vi "Methods_Insert Dividers.vi"(11 "Methods[] In":T1(array[cluster])) -> (3 "Methods[] Out":T1(array[cluster]))   [LabVIEW 2023] (continued)
name (localized)"="Convert To FlatSeq", "Long name (localized)"="Convert To Flat Sequence"}, "Method Flags"={"IsDeprecated"=FALSE, "IsPrivate"=FALSE, "IsScripting"=TRUE, "IsNotInRun-Time"=FALSE}, "Divider"=FALSE}, {"Class Info"={"Unique ID string"="16408", "Parent ID string"="16406", "Class Name (unlocalized)"="CaseStructure", "Class Name (localized)"="CaseStructure"}, "Method Info"={"Unique ID string"="6364c00", "Data name"="Remove Empty Cases", "Short name (localized)"="Remove Empty Cases", "Long name (localized)"="Remove Empty Cases"}, "Method Flags"={"IsDeprecated"=FALSE, "IsPrivate"=FALSE, "IsScripting"=TRUE, "IsNotInRun-Time"=TRUE}, "Divider"=FALSE}, {"Class Info"={"Unique ID string"="16408", "Parent ID string"="16406", "Class Name (unlocalized)"="CaseStructure", "Class Name (localized)"="CaseStructure"}, "Method Info"={"Unique ID string"="6364c02", "Data name"="SetDefaultCase", "Short name (localized)"="SetDefaultCase", "Long name (localized)"="Set Default Case"}, "Method Flags"={"IsDeprecated"=FALSE, "IsPrivate"=FALSE, "IsScripting"=TRUE, "IsNotInRun-Time"=TRUE}, "Divider"=FALSE}, {"Class Info"={"Unique ID string"="16408", "Parent ID string"="16406", "Class Name (unlocalized)"="CaseStructure", "Class Name (localized)"="CaseStructure"}, "Method Info"={"Unique ID string"="6364c03", "Data name"="RemoveDefault", "Short name (localized)"="RemoveDefault", "Long name (localized)"="Remove Default"}, "Method Flags"={"IsDeprecated"=FALSE, "IsPrivate"=FALSE, "IsScripting"=TRUE, "IsNotInRun-Time"=TRUE}, "Divider"=FALSE}, {"Class Info"={"Unique ID string"="16408", "Parent ID string"="16406", "Class Name (unlocalized)"="CaseStructure", "Class Name (localized)"="CaseStructure"}, "Method Info"={"Unique ID string"="6364c04", "Data name"="GetFrameIndex", "Short name (localized)"="GetFrameIndex", "Long name (localized)"="Get Frame Index"}, "Method Flags"={"IsDeprecated"=FALSE, "IsPrivate"=FALSE, "IsScripting"=TRUE, "IsNotInRun-Time"=FALSE}, "Divider"=FALSE}, {"Class Info"={"Unique ID string"="16409", "Parent ID string"="16421", "Class Name (unlocalized)"="Formula", "Class Name (localized)"="Formula"}, "Method Info"={"Unique ID string"="6365800", "Data name"="Add Input", "Short name (localized)"="Add Input", "Long name (localized)"="Add Input"}, "Method Flags"={"IsDeprecated"=FALSE, "IsPrivate"=FALSE, "IsScripting"=TRUE, "IsNotInRun-Time"=TRUE}, "Divider"=FALSE}, {"Class Info"={"Unique ID string"="16409", "Parent ID string"="16421", "Class Name (unlocalized)"="Formula", "Class Name (localized)"="Formula"}, "Method Info"={"Unique ID string"="6365801", "Data name"="Add Output", "Short name (localized)"="Add Output", "Long name (localized)"="Add Output"}, "Method Flags"={"IsDeprecated"=FALSE, "IsPrivate"=FALSE, "IsScripting"=TRUE, "IsNotInRun-Time"=TRUE}, "Divider"=FALSE}, {"Class Info"={"Unique ID string"="16410", "Parent ID string"="16421", "Class Name (unlocalized)"="GrowableFunction", "Class Name (localized)"="GrowableFunction"}, "Method Info"={"Unique ID string"="6367c01", "Data name"="Resize.AddChunk", "Short name (localized)"="Resize.AddChunk", "Long name (localized)"="Resize:Add Chunk"}, "Method Flags"={"IsDeprecated"=FALSE, "IsPrivate"=FALSE, "IsScripting"=TRUE, "IsNotInRun-Time"=TRUE}, "Divider"=FALSE}, {"Class Info"={"Unique ID string"="16410", "Parent ID string"="16421", "Class Name (unlocalized)"="GrowableFunction", "Class Name (localized)"="GrowableFunction"}, "Method Info"={"Unique ID string"="6367c02", "Data name"="Resize.RemoveChunk", "Short name (localized)"="Resize.RemoveChunk", "Long name (localized)"="Resize:Remove Chunk"}, "Method Flags"={"IsDeprecated"=FALSE, "IsPrivate"=FALSE, "IsScripting"=TRUE, "IsNotInRun-Time"=TRUE}, "Divider"=FALSE}, {"Class Info"={"Unique ID string"="16416", "Parent ID string"="16410", "Class Name (unlocalized)"="CIN", "Class Name (localized)"="CIN"}, "Method Info"={"Unique ID string"="636c400", "Data name"="Load Code Resource", "Short name (localized)"="Load Code Resource", "Long name (localized)"="Load Code Resource"}, "Method Flags"={"IsDeprecated"=FALSE, "IsPrivate"=FALSE, "IsScripting"=TRUE, "IsNotInRun-Time"=TRUE}, "Divider"=FALSE}, {"Class Info"={"Unique ID string"="16416", "Parent ID string"="16410", "Class Name (unlocalized)"="CIN", "Class Name (localized)"="CIN"}, "Method Info"={"Unique ID string"="636c401", "Data name"="Create C File", "Short name (localized)"="Create C File", "Long name (localized)"="Create C File"}, "Method Flags"={"IsDeprecated"=FALSE, "IsPrivate"=FALSE, "IsScripting"=TRUE, "IsNotInRun-Time"=TRUE}, "Divider"=FALSE}, {"Class Info"={"Unique ID string"="16416", "Parent ID string"="16410", "Class Name (unlocalized)"="CIN", "Class Name (localized)"="CIN"}, "Method Info"={"Unique ID string"="636c402", "Data name"="AddParameterAfter", "Short name (localized)"="AddParameterAfter", "Long name (localized)"="Add Parameter After"}, "Method Flags"={"IsDeprecated"=FALSE, "IsPrivate"=FALSE, "IsScripting"=TRUE, "IsNotInRun-Time"=FALSE}, "Divider"=FALSE}, {"Class Info"={"Unique ID string"="16416", "Parent ID string"="16410", "Class Name (unlocalized)"="CIN", "Class Name (localized)"="CIN"}, "Method Info"={"Unique ID string"="636c403", "Data name"="RemoveParameter", "Short name (localized)"="RemoveParameter", "Long name (localized)"="Remove Parameter"}, "Method Flags"={"IsDeprecated"=FALSE, "IsPrivate"=FALSE, "IsScripting"=TRUE, "IsNotInRun-Time"=FALSE}, "Divider"=FALSE}, {"Class Info"={"Unique ID string"="16416", "Parent ID string"="16410", "Class Name (unlocalized)"="CIN", "Class Name (localized)"="CIN"}, "Method Info"={"Unique ID string"="636c404", "Data name"="PurgeCodeResource", "Short name (localized)"="PurgeCodeResource", "Long name (localized)"="Purge Code Resource"}, "Method Flags"={"IsDeprecated"=FALSE, "IsPrivate"=FALSE, "IsScripting"=TRUE, "IsNotInRun-Time"=FALSE}, "Divider"=FALSE}, {"Class Info"={"Unique ID string"="16417", "Parent ID string"="16410", "Class Name (unlocalized)"="CallLibrary", "Class Name (localized)"="CallLibrary"}, "Method Info"={"Unique ID string"="636d000", "Data name"="Prototype", "Short name (localized)"="Prototype", "Long name (localized)"="Prototype"}, "Method Flags"={"IsDeprecated"=FALSE, "IsPrivate"=FALSE, "IsScripting"=TRUE, "IsNotInRun-Time"=TRUE}, "Divider"=FALSE}, {"Class Info"={"Unique ID string"="16417", "Parent ID string"="16410", "Class Name (unlocalized)"="CallLibrary", "Class Name (localized)"="CallLibrary"}, "Method Info"={"Unique ID string"="636d001", "Data name"="CreateCFile", "Short name (localized)"="CreateCFile", "Long name (localized)"="Create C File"}, "Method Flags"={"IsDeprecated"=FALSE, "IsPrivate"=FALSE, "IsScripting"=TRUE, "IsNotInRun-Time"=FALSE}, "Divider"=FALSE}, {"Class Info"={"Unique ID string"="16417", "Parent ID string"="16410", "Class Name (unlocalized)"="CallLibrary", "Class Name (localized)"="CallLibrary"}, "Method Info"={"Unique ID string"="636d002", "Data name"="TypeOnlyParam", "Short name (localized)"="TypeOnlyParam", "Long name (localized)"="Type Only Param"}, "Method Flags"={"IsDeprecated"=FALSE, "IsPrivate"=TRUE, "IsScripting"=TRUE, "IsNotInRun-Time"=FALSE}, "Divider"=FALSE}, {"Class Info"={"Unique ID string"="16419", "Parent ID string"="16418", "Class Name (unlocalized)"="Property", "Class Name (localized)"="Property"}, "Method Info"={"Unique ID string"="636f400", "Data name"="Get Prop Item", "Short name (localized)"="Get Prop Item", "Long name (localized)"="Get Property Item"}, "Method Flags"={"IsDeprecated"=FALSE, "IsPrivate"=FALSE, "IsScripting"=TRUE, "IsNotInRun-Time"=TRUE}, "Divider"=FALSE}, {"Class Info"={"Unique ID string"="16419", "Parent ID string"="16418", "Class Name (unlocalized)"="Property", "Class Name (localized)"="Property"}, "Method Info"={"Unique ID string"="636f401", "Data name"="AddPropertyItemAfter", "Short name (localized)"="AddPropertyItemAfter", "Long name (localized)"="Add Property Item After"}, "Method Flags"={"IsDeprecated"=FALSE, "IsPrivate"=FALSE, "IsScripting"=TRUE, "IsNotInRun-Time"=FALSE}, "Divider"=FALSE}, {"Class Info"={"Unique ID string"="16419", "Parent ID string"="16418", "Class Name (unlocalized)"="Property", "Class Name (localized)"="Property"}, "Method Info"={"Unique ID string"="636f402", "Data name"="RemovePropertyItem", "Short name (localized)"="RemovePropertyItem", "Long name (localized)"="Remove Property Item"}, "Method Flags"={"IsDeprecated"=FALSE, "IsPrivate"=FALSE, "IsScripting"=TRUE, "IsNotInRun-Time"=FALSE}, "Divider"=FALSE}, {"Class Info"={"Unique ID string"="16419", "Parent ID string"="16418", "Class Name (unlocalized)"="Property", "Class Name (localized)"="Property"}, "Method Info"={"Unique ID string"="636f403", "Data name"="LinkToControl", "Short name (localized)"="LinkToControl", "Long name (localized)"="Link To Control"}, "Method Flags"={"IsDeprecated"=FALSE, "IsPrivate"=FALSE, "IsScripting"=TRUE, "IsNotInRun-Time"=FALSE}, "Divider"=FALSE}, {"Class Info"={"Unique ID string"="16419", "Parent ID string"="16418", "Class Name (unlocalized)"="Property", "Class Name (localized)"="Property"}, "Method Info"={"Unique ID string"="636f404", "Data name"="DisconnectFromControl", "Short name (localized)"="DisconnectFromControl", "Long name (localized)"="Disconnect From Control"}, "Method Flags"={"IsDeprecated"=FALSE, "IsPrivate"=FALSE, "IsScripting"=TRUE, "IsNotInRun-Time"=FALSE}, "Divider"=FALSE}, {"Class Info"={"Unique ID string"="16419", "Parent ID string"="16418", "Class Name (unlocalized)"="Property", "Class Name (localized)"="Property"}, "Method Info"={"Unique ID string"="636f405", "Data name"="SetProperties[]", "Short name (localized)"="SetProperties[]", "Long name (localized)"="Set Properties[]"}, "Method Flags"={"IsDeprecated"=FALSE, "IsPrivate"=FALSE, "IsScripting"=TRUE, "IsNotInRun-Time"=TRUE}, "Divider"=FALSE}, {"Class Info"={"Unique ID string"="16419", "Parent ID string"="16418", "Class Name (unlocalized)"="Property", "Class Name (localized)"="Property"}, "Method Info"={"Unique ID string"="636f406", "Data name"="SetProperties_AllowPrivate", "Short name (localized)"="SetProperties_AllowPrivate", "Long name (localized)"="Set Properties[] (Allow Private)"}, "Method Flags"={"IsDeprecated"=FALSE, "IsPrivate"=TRUE, "IsScripting"=TRUE, "IsNotInRun-Time"=TRUE}, "Divider"=FALSE}, {"Class Info"={"Unique ID string"="16420", "Parent ID string"="16418", "Class Name (unlocalized)"="Invoke", "Class Name (localized)"="Invoke"}, "Method Info"={"Unique ID string"="6370000", "Data name"="LinkToControl", "Short name (localized)"="LinkToControl", "Long name (localized)"="Link To Control"}, "Method Flags"={"IsDeprecated"=FALSE, "IsPrivate"=FALSE, "IsScripting"=TRUE, "IsNotInRun-Time"=FALSE}, "Divider"=FALSE}, {"Class Info"={"Unique ID string"="16420", "Parent ID string"="16418", "Class Name (unlocalized)"="Invoke", "Class Name (localized)"="Invoke"}, "Method Info"={"Unique ID string"="6370001", "Data name"="DisconnectFromControl", "Short name (localized)"="DisconnectFromControl", "Long name (localized)"="Disconnect From Control"}, "Method Flags"={"IsDeprecated"=FALSE, "IsPrivate"=FALSE, "IsScripting"=TRUE, "IsNotInRun-Time"=FALSE}, "Divider"=FALSE}, {"Class Info"={"Unique ID string"="16420", "Parent ID string"="16418", "Class Name (unlocalized)"="Invoke", "Class Name (localized)"="Invoke"}, "Method Info"={"Unique ID string"="6370002", "Data name"="SetMethod", "Short name (localized)"="SetMethod", "Long name (localized)"="Set Method"}, "Method Flags"={"IsDeprecated"=FALSE, "IsPrivate"=FALSE, "IsScripting"=TRUE, "IsNotInRun-Time"=TRUE}, "Divider"=FALSE}, {"Class Info"={"Unique ID string"="16420", "Parent ID string"="16418", "Class Name (unlocalized)"="Invoke", "Class Name (localized)"="Invoke"}, "Method Info"={"Unique ID string"="6370003", "Data name"="SetMethod_AllowPrivate", "Short name (localized)"="SetMethod_AllowPrivate", "Long name (localized)"="Set Method (Allow Private)"}, "Method Flags"={"IsDeprecated"=FALSE, "IsPrivate"=TRUE, "IsScripting"=TRUE, "IsNotInRun-Time"=TRUE}, "Divider"=FALSE}, {"Class Info"={"Unique ID string"="16421", "Parent ID string"="36", "Class Name (unlocalized)"="Node", "Class Name (localized)"="Node"}, "Method Info"={"Unique ID string"="6358c00", "Data name"="Connect Wires", "Short name (localized)"="Connect Wires", "Long name (localized)"="Connect Wires"}, "Method Flags"={"IsDeprecated"=FALSE, "IsPrivate"=FALSE, "IsScripting"=TRUE, "IsNotInRun-Time"=TRUE}, "Divider"=FALSE}, {"Class Info"={"Unique ID string"="16421", "Parent ID string"="36", "Class Name (unlocalized)"="Node", "Class Name (localized)"="Node"}, "Method Info"={"Unique ID string"="6358c01", "Data name"="Get Image", "Short name (localized)"="Get Image", "Long name (localized)"="Get Image"}, "Method Flags"={"IsDeprecated"=FALSE, "IsPrivate"=FALSE, "IsScripting"=TRUE, "IsNotInRun-Time"=TRUE}, "Divider"=FALSE}, {"Class Info"={"Unique ID string"="16423", "Parent ID string"="16384", "Class Name (unlocalized)"="TopLevelDiagram", "Class Name (localized)"="TopLevelDiagram"}, "Method Info"={"Unique ID string"="6349001", "Data name"="Clear Selection", "Short name (localized)"="Clear Selection", "Long name (localized)"="Clear Selection"}, "Method Flags"={"IsDeprecated"=FALSE, "IsPrivate"=FALSE, "IsScripting"=TRUE, "IsNotInRun-Time"=TRUE}, "Divider"=FALSE}, {"Class Info"={"Unique ID string"="16423", "Parent ID string"="16384", "Class Name (unlocalized)"="TopLevelDiagram", "Class Name (localized)"="TopLevelDiagram"}, "Method Info"={"Unique ID string"="6349002", "Data name"="Make Selection", "Short name (localized)"="Make Selection", "Long name (localized)"="Make Selection"}, "Method Flags"={"IsDeprecated"=FALSE, "IsPrivate"=FALSE, "IsScripting"=TRUE, "IsNotInRun-Time"=TRUE}, "Divider"=FALSE}, {"Class Info"={"Unique ID string"="16423", "Parent ID string"="16384", "Class Name (unlocalized)"="TopLevelDiagram", "Class Name (localized)"="TopLevelDiagram"}, "Method Info"={"Unique ID string"="6349003", "Data name"="Copy Selection", "Short name (localized)"="Copy Selection", "Long name (localized)"="Copy Selection"}, "Method Flags"={"IsDeprecated"=FALSE, "IsPrivate"=FALSE, "IsScripting"=TRUE, "IsNotInRun-Time"=TRUE}, "Divider"=FALSE}, {"Class Info"={"Unique ID string"="16423", "Parent ID string"="16384", "Class Name (unlocalized)"="TopLevelDiagram", "Class Name (localized)"="TopLevelDiagram"}, "Method Info"={"Unique ID string"="6349004", "Data name"="CutSelection", "Short name (localized)"="CutSelection", "Long name (localized)"="Cut Selection"}, "Method Flags"={"IsDeprecated"=FALSE, "IsPrivate"=FALSE, "IsScripting"=TRUE, "IsNotInRun-Time"=FALSE}, "Divider"=FALSE}, {"Class Info"={"Unique ID string"="16423", "Parent ID string"="16384", "Class Name (unlocalized)"="TopLevelDiagram", "Class Name (localized)"="TopLevelDiagram"}, "Method Info"={"Unique ID string"="6349005", "Data name"="MakeSelectionFromRect", "Short name (localized)"="MakeSelectionFromRect", "Long name (localized)"="Make Selection From Rect"}, "Method Flags"={"IsDeprecated"=FALSE, "IsPrivate"=FALSE, "IsScripting"=TRUE, "IsNotInRun-Time"=FALSE}, "Divider"=FALSE}, {"Class Info"={"Unique ID string"="16423", "Parent ID string"="16384", "Class Name (unlocalized)"="TopLevelDiagram", "Class Name (localized)"="TopLevelDiagram"}, "Method Info"={"Unique ID string"="6349006", "Data name"="AlignSelection", "Short name (localized)"="AlignSelection", "Long name (localized)"="Align Selection"}, "Method Flags"={"IsDeprecated"=FALSE, "IsPrivate"=FALSE, "IsScripting"=TRUE, "IsNotInRun-Time"=FALSE}, "Divider"=FALSE}, {"Class Info"={"Unique ID string"="16423", "Parent ID string"="16384", "Class Name (unlocalized)"="TopLevelDiagram", "Class Name (localized)"="TopLevelDiagram"}, "Method Info"={"Unique ID string"="6349007", "Data name"="DistributeSelection", "Short name (localized)"="DistributeSelection", "Long name (localized)"="Distribute Selection"}, "Method Flags"={"IsDeprecated"=FALSE, "IsPrivate"=FALSE, "IsScripting"=TRUE, "IsNotInRun-Time"=FALSE}, "Divider"=FALSE}, {"Class Info"={"Unique ID string"="16423", "Parent ID string"="16384", "Class Name (unlocalized)"="TopLevelDiagram", "Class Name (localized)"="TopLevelDiagram"}, "Method Info"={"Unique ID string"="6349008", "Data name"="MoveSelectionToFront", "Short name (localized)"="MoveSelectionToFront", "Long name (localized)"="Move Selection To Front"}, "Method Flags"={"IsDeprecated"=FALSE, "IsPrivate"=FALSE, "IsScripting"=TRUE, "IsNotInRun-Time"=FALSE}, "Divider"=FALSE}, {"Class Info"={"Unique ID string"="16423", "Parent ID string"="16384", "Class Name (unlocalized)"="TopLevelDiagram", "Class Name (localized)"="TopLevelDiagram"}, "Method Info"={"Unique ID string"="6349009", "Data name"="MoveSelectionToBack", "Short name (localized)"="MoveSelectionToBack", "Long name (localized)"="Move Selection To Back"}, "Method Flags"={"IsDeprecated"=FALSE, "IsPrivate"=FALSE, "IsScripting"=TRUE, "IsNotInRun-Time"=FALSE}, "Divider"=FALSE}, {"Class Info"={"Unique ID string"="16423", "Parent ID string"="16384", "Class Name (unlocalized)"="TopLevelDiagram", "Class Name (localized)"="TopLevelDiagram"}, "Method Info"={"Unique ID string"="634900a", "Data name"="MoveSelectionForward", "Short name (localized)"="MoveSelectionForward", "Long name (localized)"="Move Selection Forward"}, "Method Flags"={"IsDeprecated"=FALSE, "IsPrivate"=FALSE, "IsScripting"=TRUE, "IsNotInRun-Time"=FALSE}, "Divider"=FALSE}, {"Class Info"={"Unique ID string"="16423", "Parent ID string"="16384", "Class Name (unlocalized)"="TopLevelDiagram", "Class Name (localized)"="TopLevelDiagram"}, "Method Info"={"Unique ID string"="634900b", "Data name"="MoveSelectionBackward", "Short name (localized)"="MoveSelectionBackward", "Long name (localized)"="Move Selection Backward"}, "Method Flags"={"IsDeprecated"=FALSE, "IsPrivate"=FALSE, "IsScripting"=TRUE, "IsNotInRun-Time"=FALSE}, "Divider"=FALSE}, {"Class Info"={"Unique ID string"="16423", "Parent ID string"="16384", "Class Name (unlocalized)"="TopLevelDiagram", "Class Name (localized)"="TopLevelDiagram"}, "Method Info"={"Unique ID string"="634900c", "Data name"="RemoveFromSelection", "Short name (localized)"="RemoveFromSelection", "Long name (localized)"="RemoveFromSelection"}, "Method Flags"={"IsDeprecated"=FALSE, "IsPrivate"=FALSE, "IsScripting"=TRUE, "IsNotInRun-Time"=TRUE}, "Divider"=FALSE}, {"Class Info"={"Unique ID string"="16423", "Parent ID string"="16384", "Class Name (unlocalized)"="TopLevelDiagram", "Class Name (localized)"="TopLevelDiagram"}, "Method Info"={"Unique ID string"="634900e", "Data name"="NewVIFromSelection", "Short name (localized)"="NewVIFromSelection", "Long name (localized)"="NewVIFromSelection"}, "Method Flags"={"IsDeprecated"=FALSE, "IsPrivate"=TRUE, "IsScripting"=TRUE, "IsNotInRun-Time"=FALSE}, "Divider"=FALSE}, {"Class Info"={"Unique ID string"="16423", "Parent ID string"="16384", "Class Name (unlocalized)"="TopLevelDiagram", "Class Name (localized)"="TopLevelDiagram"}, "Method Info"={"Unique ID string"="634900f", "Data name"="Move Selected Objects", "Short name (localized)"="Move Selected Objects", "Long name (localized)"="Move Selected Objects"}, "Method Flags"={"IsDeprecated"=FALSE, "IsPrivate"=FALSE, "IsScripting"=TRUE, "IsNotInRun-Time"=FALSE}, "Divider"=FALSE}, {"Class Info"={"Unique ID string"="16423", "Parent ID string"="16384", "Class Name (unlocalized)"="TopLevelDiagram", "Class Name (localized)"="TopLevelDiagram"}, "Method Info"={"Unique ID string"="6349010", "Data name"="EncloseSelection2", "Short name (localized)"="EncloseSelection2", "Long name (localized)"="Enclose Selection 2"}, "Method Flags"={"IsDeprecated"=FALSE, "IsPrivate"=FALSE, "IsScripting"=TRUE, "IsNotInRun-Time"=FALSE}, "Divider"=FALSE}, {"Class Info"={"Unique ID string"="16423", "Parent ID string"="16384", "Class Name (unlocalized)"="TopLevelDiagram", "Class Name (localized)"="TopLevelDiagram"}, "Method Info"={"Unique ID string"="6349011", "Data name"="ExternalEditorWizard", "Short name (localized)"="ExternalEditorWizard", "Long name (localized)"="External Editor Wizard"}, "Method Flags"={"IsDeprecated"=FALSE, "IsPrivate"=FALSE, "IsScripting"=TRUE, "IsNotInRun-Time"=FALSE}, "Divider"=FALSE}, {"Class Info"={"Unique ID string"="16435", "Parent ID string"="16405", "Class Name (unlocalized)"="WhileLoop", "Class Name (localized)"="WhileLoop"}, "Method Info"={"Unique ID string"="6362800", "Data name"="Replace With TimeLoop", "Short name (localized)"="Replace With TimeLoop", "Long name (localized)"="Replace With TimeLoop"}, "Method Flags"={"IsDeprecated"=FALSE, "IsPrivate"=FALSE, "IsScripting"=TRUE, "IsNotInRun-Time"=FALSE}, "Divider"=FALSE}, {"Class Info"={"Unique ID string"="16439", "Parent ID string"="36", "Class Name (unlocalized)"="Wire", "Class Name (localized)"="Wire"}, "Method Info"={"Unique ID string"="6370c00", "Data name"="AttachProbe", "Short name (localized)"="AttachProbe", "Long name (localized)"="Attach Probe"}, "Method Flags"={"IsDeprecated"=FALSE, "IsPrivate"=FALSE, "IsScripting"=TRUE, "IsNotInRun-Time"=TRUE}, "Divider"=FALSE}, {"Class Info"={"Unique ID string"="16439", "Parent ID string"="36", "Class Name (unlocalized)"="Wire", "Class Name (localized)"="Wire"}, "Method Info"={"Unique ID string"="6370c01", "Data name"="Remove Probe", "Short name (localized)"="Remove Probe", "Long name (localized)"="Remove Probe"}, "Method Flags"={"IsDeprecated"=FALSE, "IsPrivate"=FALSE, "IsScripting"=TRUE, "IsNotInRun-Time"=TRUE}, "Divider"=FALSE}, {"Class Info"={"Unique ID string"="16439", "Parent ID string"="36", "Class Name (unlocalized)"="Wire", "Class Name (localized)"="Wire"}, "Method Info"={"Unique ID string"="6370c02", "Data name"="Create Constant", "Short name (localized)"="Create Constant", "Long name (localized)"="Create Constant (Not Implemented)"}, "Method Flags"={"IsDeprecated"=FALSE, "IsPrivate"=TRUE, "IsScripting"=TRUE, "IsNotInRun-Time"=TRUE}, "Divider"=FALSE}, {"Class Info"={"Unique ID string"="16439", "Parent ID string"="36", "Class Name (unlocalized)"="Wire", "Class Name (localized)"="Wire"}, "Method Info"={"Unique ID string"="6370c03", "Data name"="Create Control", "Short name (localized)"="Create Control", "Long name (localized)"="Create Control (Not Implemented)"}, "Method Flags"={"IsDeprecated"=FALSE, "IsPrivate"=TRUE, "IsScripting"=TRUE, "IsNotInRun-Time"=TRUE}, "Divider"=FALSE}, {"Class Info"={"Unique ID string"="16439", "Parent ID string"="36", "Class Name (unlocalized)"="Wire", "Class Name (localized)"="Wire"}, "Method Info"={"Unique ID string"="6370c04", "Data name"="Create Indicator", "Short name (localized)"="Create Indicator", "Long name (localized)"="Create Indicator (Not Implemented)"}, "Method Flags"={"IsDeprecated"=FALSE, "IsPrivate"=TRUE, "IsScripting"=TRUE, "IsNotInRun-Time"=TRUE}, "Divider"=FALSE}, {"Class Info"={"Unique ID string"="16439", "Parent ID string"="36", "Class Name (unlocalized)"="Wire", "Class Name (localized)"="Wire"}, "Method Info"={"Unique ID string"="6370c05", "Data name"="CleanUpWire", "Short name (localized)"="CleanUpWire", "Long name (localized)"="Clean Up Wire"}, "Method Flags"={"IsDeprecated"=FALSE, "IsPrivate"=FALSE, "IsScripting"=TRUE, "IsNotInRun-Time"=FALSE}, "Divider"=FALSE}, {"Class Info"={"Unique ID string"="16439", "Parent ID string"="36", "Class Name (unlocalized)"="Wire", "Class Name (localized)"="Wire"}, "Method Info"={"Unique ID string"="6370c06", "Data name"="Insert Node", "Short name (localized)"="Insert Node", "Long name (localized)"="Insert Node"}, "Method Flags"={"IsDeprecated"=FALSE, "IsPrivate"=FALSE, "IsScripting"=TRUE, "IsNotInRun-Time"=TRUE}, "Divider"=FALSE}, {"Class Info"={"Unique ID string"="16439", "Parent ID string"="36", "Class Name (unlocalized)"="Wire", "Class Name (localized)"="Wire"}, "Method Info"={"Unique ID string"="6370c07", "Data name"="CopyProbesToCompanion", "Short name (localized)"="CopyProbesToCompanion", "Long name (localized)"="Copy Probes To Companion"}, "Method Flags"={"IsDeprecated"=FALSE, "IsPrivate"=FALSE, "IsScripting"=TRUE, "IsNotInRun-Time"=FALSE}, "Divider"=FALSE}, {"Class Info"={"Unique ID string"="16439", "Parent ID string"="36", "Class Name (unlocalized)"="Wire", "Class Name (localized)"="Wire"}, "Method Info"={"Unique ID string"="6370c08", "Data name"="RemoveLooseEnds", "Short name (localized)"="RemoveLooseEnds", "Long name (localized)"="Remove Loose Ends"}, "Method Flags"={"IsDeprecated"=FALSE, "IsPrivate"=FALSE, "IsScripting"=TRUE, "IsNotInRun-Time"=FALSE}, "Divider"=FALSE}, {"Class Info"={"Unique ID string"="16439", "Parent ID string"="36", "Class Name (unlocalized)"="Wire", "Class Name (localized)"="Wire"}, "Method Info"={"Unique ID string"="6370c09", "Data name"="Insert Node By Ref", "Short name (localized)"="Insert Node By Ref", "Long name (localized)"="Insert Node By Ref (Not Implemented)"}, "Method Flags"={"IsDeprecated"=FALSE, "IsPrivate"=TRUE, "IsScripting"=TRUE, "IsNotInRun-Time"=TRUE}, "Divider"=FALSE}, {"Class Info"={"Unique ID string"="16439", "Parent ID string"="36", "Class Name (unlocalized)"="Wire", "Class Name (localized)"="Wire"}, "Method Info"={"Unique ID string"="6370c0a", "Data name"="GetErrorList", "Short name (localized)"="GetErrorList", "Long name (localized)"="Get Error List"}, "Method Flags"={"IsDeprecated"=FALSE, "IsPrivate"=TRUE, "IsScripting"=TRUE, "IsNotInRun-Time"=FALSE}, "Divider"=FALSE}, {"Class Info"={"Unique ID string"="16439", "Parent ID string"="36", "Class Name (unlocalized)"="Wire", "Class Name (localized)"="Wire"}, "Method Info"={"Unique ID string"="6370c0b", "Data name"="DeleteJoint", "Short name (localized)"="DeleteJoint", "Long name (localized)"="Delete Joint"}, "Method Flags"={"IsDeprecated"=FALSE, "IsPrivate"=FALSE, "IsScripting"=TRUE, "IsNotInRun-Time"=FALSE}, "Divider"=FALSE}, {"Class Info"={"Unique ID string"="16439", "Parent ID string"="36", "Class Name (unlocalized)"="Wire", "Class Name (localized)"="Wire"}, "Method Info"={"Unique ID string"="6370c0c", "Data name"="AttachSmplingProbe", "Short name (localized)"="AttachSmplingProbe", "Long name (localized)"="Attach Sampling Probe"}, "Method Flags"={"IsDeprecated"=FALSE, "IsPrivate"=TRUE, "IsScripting"=TRUE, "IsNotInRun-Time"=TRUE}, "Divider"=FALSE}, {"Class Info"={"Unique ID string"="16439", "Parent ID string"="36", "Class Name (unlocalized)"="Wire", "Class Name (localized)"="Wire"}, "Method Info"={"Unique ID string"="6370c0d", "Data name"="DisconnectTerminal", "Short name (localized)"="DisconnectTerminal", "Long name (localized)"="Disconnect Terminal"}, "Method Flags"={"IsDeprecated"=FALSE, "IsPrivate"=FALSE, "IsScripting"=TRUE, "IsNotInRun-Time"=TRUE}, "Divider"=FALSE}, {"Class Info"={"Unique ID string"="16442", "Parent ID string"="16426", "Class Name (unlocalized)"="LeftShiftRegister", "Class Name (localized)"="LeftShiftRegister"}, "Method Info"={"Unique ID string"="6374800", "Data name"="AddElem", "Short name (localized)"="AddElem", "Long name (localized)"="Add Element"}, "Method Flags"={"IsDeprecated"=FALSE, "IsPrivate"=FALSE, "IsScripting"=TRUE, "IsNotInRun-Time"=TRUE}, "Divider"=FALSE}, {"Class Info"={"Unique ID string"="16444", "Parent ID string"="36", "Class Name (unlocalized)"="PropertyItem", "Class Name (localized)"="PropertyItem"}, "Method Info"={"Unique ID string"="6de8d801", "Data name"="SetProperty", "Short name (localized)"="SetProperty", "Long name (localized)"="Set Property"}, "Method Flags"={"IsDeprecated"=FALSE, "IsPrivate"=FALSE, "IsScripting"=TRUE, "IsNotInRun-Time"=FALSE}, "Divider"=FALSE}, {"Class Info"={"Unique ID string"="16444", "Parent ID string"="36", "Class Name (unlocalized)"="PropertyItem", "Class Name (localized)"="PropertyItem"}, "Method Info"={"Unique ID string"="6de8d802", "Data name"="SetProperty_AllowPrivate", "Short name (localized)"="SetProperty_AllowPrivate", "Long name (localized)"="Set Property (Allow Private)"}, "Method Flags"={"IsDeprecated"=FALSE, "IsPrivate"=TRUE, "IsScripting"=TRUE, "IsNotInRun-Time"=TRUE}, "Divider"=FALSE}, {"Class Info"={"Unique ID string"="16448", "Parent ID string"="16445", "Class Name (unlocalized)"="VISAResourceNameConstant", "Class Name (localized)"="VISAResourceNameConstant"}, "Method Info"={"Unique ID string"="43106c00", "Data name"="SetClassName", "Short name (localized)"="SetClassName", "Long name (localized)"="Set Class Name"}, "Method Flags"={"IsDeprecated"=FALSE, "IsPrivate"=TRUE, "IsScripting"=TRUE, "IsNotInRun-Time"=FALSE}, "Divider"=FALSE}, {"Class Info"={"Unique ID string"="16449", "Parent ID string"="16445", "Class Name (unlocalized)"="IVILogicalNameConstant", "Class Name (localized)"="IVILogicalNameConstant"}, "Method Info"={"Unique ID string"="10cc2800", "Data name"="SetClassName", "Short name (localized)"="SetClassName", "Long name (localized)"="Set Class Name"}, "Method Flags"={"IsDeprecated"=FALSE, "IsPrivate"=TRUE, "IsScripting"=TRUE, "IsNotInRun-Time"=FALSE}, "Divider"=FALSE}, {"Class Info"={"Unique ID string"="16452", "Parent ID string"="16482", "Class Name (unlocalized)"="ClassSpecifierConstant", "Class Name (localized)"="ClassSpecifierConstant"}, "Method Info"={"Unique ID string"="566ef800", "Data name"="SetType", "Short name (localized)"="SetType", "Long name (localized)"="Set Type"}, "Method Flags"={"IsDeprecated"=FALSE, "IsPrivate"=FALSE, "IsScripting"=TRUE, "IsNotInRun-Time"=FALSE}, "Divider"=FALSE}, {"Class Info"={"Unique ID string"="16455", "Parent ID string"="16463", "Class Name (unlocalized)"="StateDiagramWizard", "Class Name (localized)"="StateDiagramWizard"}, "Method Info"={"Unique ID string"="7e9ac000", "Data name"="AddState", "Short name (localized)"="AddState", "Long name (localized)"="AddState"}, "Method Flags"={"IsDeprecated"=FALSE, "IsPrivate"=TRUE, "IsScripting"=TRUE, "IsNotInRun-Time"=TRUE}, "Divider"=FALSE}, {"Class Info"={"Unique ID string"="16455", "Parent ID string"="16463", "Class Name (unlocalized)"="StateDiagramWizard", "Class Name (localized)"="StateDiagramWizard"}, "Method Info"={"Unique ID string"="7e9ac001", "Data name"="Update State Consts", "Short name (localized)"="Update State Consts", "Long name (localized)"="Update State Constants"}, "Method Flags"={"IsDeprecated"=FALSE, "IsPrivate"=TRUE, "IsScripting"=TRUE, "IsNotInRun-Time"=TRUE}, "Divider"=FALSE}, {"Class Info"={"Unique ID string"="16455", "Parent ID string"="16463", "Class Name (unlocalized)"="StateDiagramWizard", "Class Name (localized)"="StateDiagramWizard"}, "Method Info"={"Unique ID string"="7e9ac002", "Data name"="Add New State Items", "Short name (localized)"="Add New State Items", "Long name (localized)"="Add New State Items"}, "Method Flags"={"IsDeprecated"=FALSE, "IsPrivate"=TRUE, "IsScripting"=TRUE, "IsNotInRun-Time"=TRUE}, "Divider"=FALSE}, {"Class Info"={"Unique ID string"="16455", "Parent ID string"="16463", "Class Name (unlocalized)"="StateDiagramWizard", "Class Name (localized)"="StateDiagramWizard"}, "Method Info"={"Unique ID string"="7e9ac003", "Data name"="Add New Trans Items", "Short name (localized)"="Add New Trans Items", "Long name (localized)"="Add New Transition Items"}, "Method Flags"={"IsDeprecated"=FALSE, "IsPrivate"=TRUE, "IsScripting"=TRUE, "IsNotInRun-Time"=TRUE}, "Divider"=FALSE}, {"Class Info"={"Unique ID string"="16455", "Parent ID string"="16463", "Class Name (unlocalized)"="StateDiagramWizard", "Class Name (localized)"="StateDiagramWizard"}, "Method Info"={"Unique ID string"="7e9ac004", "Data name"="Add Transition", "Short name (localized)"="Add Transition", "Long name (localized)"="Add Transition"}, "Method Flags"={"IsDeprecated"=FALSE, "IsPrivate"=TRUE, "IsScripting"=TRUE, "IsNotInRun-Time"=TRUE}, "Divider"=FALSE}, {"Class Info"={"Unique ID string"="16455", "Parent ID string"="16463", "Class Name (unlocalized)"="StateDiagramWizard", "Class Name (localized)"="StateDiagramWizard"}, "Method Info"={"Unique ID string"="7e9ac005", "Data name"="Remove Trans", "Short name (localized)"="Remove Trans", "Long name (localized)"="Remove Transition"}, "Method Flags"={"IsDeprecated"=FALSE, "IsPrivate"=TRUE, "IsScripting"=TRUE, "IsNotInRun-Time"=TRUE}, "Divider"=FALSE}, {"Class Info"={"Unique ID string"="16455", "Parent ID string"="16463", "Class Name (unlocalized)"="StateDiagramWizard", "Class Name (localized)"="StateDiagramWizard"}, "Method Info"={"Unique ID string"="7e9ac006", "Data name"="Remove State", "Short name (localized)"="Remove State", "Long name (localized)"="Remove State"}, "Method Flags"={"IsDeprecated"=FALSE, "IsPrivate"=FALSE, "IsScripting"=TRUE, "IsNotInRun-Time"=TRUE}, "Divider"=FALSE}, {"Class Info"={"Unique ID string"="16455", "Parent ID string"="16463", "Class Name (unlocalized)"="StateDiagramWizard", "Class Name (localized)"="StateDiagramWizard"}, "Method Info"={"Unique ID string"="7e9ac007", "Data name"="Add Init Items", "Short name (localized)"="Add Init Items", "Long name (localized)"="Add Init Items"}, "Method Flags"={"IsDeprecated"=FALSE, "IsPrivate"=TRUE, "IsScripting"=TRUE, "IsNotInRun-Time"=TRUE}, "Divider"=FALSE}, {"Class Info"={"Unique ID string"="16455", "Parent ID string"="16463", "Class Name (unlocalized)"="StateDiagramWizard", "Class Name (localized)"="StateDiagramWizard"}, "Method Info"={"Unique ID string"="7e9ac00a", "Data name"="SetVisTrans", "Short name (localized)"="SetVisTrans", "Long name (localized)"="Set Vis. Trans."}, "Method Flags"={"IsDeprecated"=FALSE, "IsPrivate"=TRUE, "IsScripting"=TRUE, "IsNotInRun-Time"=TRUE}, "Divider"=FALSE}, {"Class Info"={"Unique ID string"="16455", "Parent ID string"="16463", "Class Name (unlocalized)"="StateDiagramWizard", "Class Name (localized)"="StateDiagramWizard"}, "Method Info"={"Unique ID string"="7e9ac00b", "Data name"="SetStateData", "Short name (localized)"="SetStateData", "Long name (localized)"="Set State Data"}, "Method Flags"={"IsDeprecated"=FALSE, "IsPrivate"=TRUE, "IsScripting"=TRUE, "IsNotInRun-Time"=TRUE}, "Divider"=FALSE}, {"Class Info"={"Unique ID string"="16455", "Parent ID string"="16463", "Class Name (unlocalized)"="StateDiagramWizard", "Class Name (localized)"="StateDiagramWizard"}, "Method Info"={"Unique ID string"="7e9ac00c", "Data name"="GetStateData", "Short name (localized)"="GetStateData", "Long name (localized)"="Get State Data"}, "Method Flags"={"IsDeprecated"=FALSE, "IsPrivate"=TRUE, "IsScripting"=TRUE, "IsNotInRun-Time"=TRUE}, "Divider"=FALSE}, {"Class Info"={"Unique ID string"="16455", "Parent ID string"="16463", "Class Name (unlocalized)"="StateDiagramWizard", "Class Name (localized)"="StateDiagramWizard"}, "Method Info"={"Unique ID string"="7e9ac00d", "Data name"="SetTransData", "Short name (localized)"="SetTransData", "Long name (localized)"="Set Trans. Data"}, "Method Flags"={"IsDeprecated"=FALSE, "IsPrivate"=TRUE, "IsScripting"=TRUE, "IsNotInRun-Time"=TRUE}, "Divider"=FALSE}, {"Class Info"={"Unique ID string"="16455", "Parent ID string"="16463", "Class Name (unlocalized)"="StateDiagramWizard", "Class Name (localized)"="StateDiagramWizard"}, "Method Info"={"Unique ID string"="7e9ac00e", "Data name"="GetTransData", "Short name (localized)"="GetTransData", "Long name (localized)"="Get Trans. Data"}, "Method Flags"={"IsDeprecated"=FALSE, "IsPrivate"=TRUE, "IsScripting"=TRUE, "IsNotInRun-Time"=TRUE}, "Divider"=FALSE}, {"Class Info"={"Unique ID string"="16455", "Parent ID string"="16463", "Class Name (unlocalized)"="StateDiagramWizard", "Class Name (localized)"="StateDiagramWizard"}, "Method Info"={"Unique ID string"="7e9ac00f", "Data name"="NumStates", "Short name (localized)"="NumStates", "Long name (localized)"="Num States"}, "Method Flags"={"IsDeprecated"=FALSE, "IsPrivate"=TRUE, "IsScripting"=TRUE, "IsNotInRun-Time"=TRUE}, "Divider"=FALSE}, {"Class Info"={"Unique ID string"="16455", "Parent ID string"="16463", "Class Name (unlocalized)"="StateDiagramWizard", "Class Name (localized)"="StateDiagramWizard"}, "Method Info"={"Unique ID string"="7e9ac010", "Data name"="NumTrans", "Short name (localized)"="NumTrans", "Long name (localized)"="Num Trans"}, "Method Flags"={"IsDeprecated"=FALSE, "IsPrivate"=TRUE, "IsScripting"=TRUE, "IsNotInRun-Time"=TRUE}, "Divider"=FALSE}, {"Class Info"={"Unique ID string"="16455", "Parent ID string"="16463", "Class Name (unlocalized)"="StateDiagramWizard", "Class Name (localized)"="StateDiagramWizard"}, "Method Info"={"Unique ID string"="7e9ac011", "Data name"="TransStateOutput", "Short name (localized)"="TransStateOutput", "Long name (localized)"="TransStateOutput"}, "Method Flags"={"IsDeprecated"=FALSE, "IsPrivate"=TRUE, "IsScripting"=TRUE, "IsNotInRun-Time"=TRUE}, "Divider"=FALSE}, {"Class Info"={"Unique ID string"="16455", "Parent ID string"="16463", "Class Name (unlocalized)"="StateDiagramWizard", "Class Name (localized)"="StateDiagramWizard"}, "Method Info"={"Unique ID string"="7e9ac012", "Data name"="ReorderTrans", "Short name (localized)"="ReorderTrans", "Long name (localized)"="Reorder Trans"}, "Method Flags"={"IsDeprecated"=FALSE, "IsPrivate"=TRUE, "IsScripting"=TRUE, "IsNotInRun-Time"=FALSE}, "Divider"=FALSE}, {"Class Info"={"Unique ID string"="16455", "Parent ID string"="16463", "Class Name (unlocalized)"="StateDiagramWizard", "Class Name (localized)"="StateDiagramWizard"}, "Method Info"={"Unique ID string"="7e9ac013", "Data name"="ToggleSubVICall", "Short name (localized)"="ToggleSubVICall", "Long name (localized)"="ToggleSubVICall"}, "Method Flags"={"IsDeprecated"=FALSE, "IsPrivate"=TRUE, "IsScripting"=TRUE, "IsNotInRun-Time"=FALSE}, "Divider"=FALSE}, {"Class Info"={"Unique ID string"="16455", "Parent ID string"="16463", "Class Name (unlocalized)"="StateDiagramWizard", "Class Name (localized)"="StateDiagramWizard"}, "Method Info"={"Unique ID string"="7e9ac014", "Data name"="LaunchEditor", "Short name (localized)"="LaunchEditor", "Long name (localized)"="LaunchEditor"}, "Method Flags"={"IsDeprecated"=FALSE, "IsPrivate"=TRUE, "IsScripting"=TRUE, "IsNotInRun-Time"=FALSE}, "Divider"=FALSE}, {"Class Info"={"Unique ID string"="16455", "Parent ID string"="16463", "Class Name (unlocalized)"="StateDiagramWizard", "Class Name (localized)"="StateDiagramWizard"}, "Method Info"={"Unique ID string"="7e9ac015", "Data name"="SetSelXNode", "Short name (localized)"="SetSelXNode", "Long name (localized)"="SetSelXNode"}, "Method Flags"={"IsDeprecated"=FALSE, "IsPrivate"=TRUE, "IsScripting"=TRUE, "IsNotInRun-Time"=TRUE}, "Divider"=FALSE}, {"Class Info"={"Unique ID string"="16455", "Parent ID string"="16463", "Class Name (unlocalized)"="StateDiagramWizard", "Class Name (localized)"="StateDiagramWizard"}, "Method Info"={"Unique ID string"="7e9ac016", "Data name"="GetSelXNode", "Short name (localized)"="GetSelXNode", "Long name (localized)"="GetSelXNode"}, "Method Flags"={"IsDeprecated"=FALSE, "IsPrivate"=TRUE, "IsScripting"=TRUE, "IsNotInRun-Time"=TRUE}, "Divider"=FALSE}, {"Class Info"={"Unique ID string"="16458", "Parent ID string"="16406", "Class Name (unlocalized)"="EventStructure", "Class Name (localized)"="EventStructure"}, "Method Info"={"Unique ID string"="5191800", "Data name"="GetEventDataNode", "Short name (localized)"="GetEventDataNode", "Long name (localized)"="Get Event Data Node"}, "Method Flags"={"IsDeprecated"=FALSE, "IsPrivate"=FALSE, "IsScripting"=TRUE, "IsNotInRun-Time"=TRUE}, "Divider"=FALSE}, {"Class Info"={"Unique ID string"="16458", "Parent ID string"="16406", "Class Name (unlocalized)"="EventStructure", "Class Name (localized)"="EventStructure"}, "Method Info"={"Unique ID string"="5191801", "Data name"="GetEventFilterNode", "Short name (localized)"="GetEventFilterNode", "Long name (localized)"="Get Event Filter Node"}, "Method Flags"={"IsDeprecated"=FALSE, "IsPrivate"=FALSE, "IsScripting"=TRUE, "IsNotInRun-Time"=TRUE}, "Divider"=FALSE}, {"Class Info"={"Unique ID string"="16458", "Parent ID string"="16406", "Class Name (unlocalized)"="EventStructure", "Class Name (localized)"="EventStructure"}, "Method Info"={"Unique ID string"="5191802", "Data name"="GetHandledEvents", "Short name (localized)"="GetHandledEvents", "Long name (localized)"="Get Handled Events"}, "Method Flags"={"IsDeprecated"=FALSE, "IsPrivate"=FALSE, "IsScripting"=TRUE, "IsNotInRun-Time"=TRUE}, "Divider"=FALSE}, {"Class Info"={"Unique ID string"="16458", "Parent ID string"="16406"
